vi "3-2 numero di valori casuali generati da RAN - ritardo controllabile da pannello.vi"(4 "stop":bool, 5 "offset":dbl=1.0 format="%.2f", 6 "mult":dbl=100.0 format="%.2f", 7 "ritardo SET":dbl=30.0 format="%.2f") -> (0 "Tempo\ntrascorso":u32, 1 "Ritardo":dbl format="%.2f", 2 "Iterazioni":dbl format="%.2f", 3 "random":dbl format="%.2f")   [LabVIEW 2012]
panel:
  out "random\ngraph":dbl(graph)
  # "Determinare il numero di valori casuali generati da RAN (VI\nche genera un numero compreso tra 1 e 101) \ndall'avvio alla pressione del tasto stop. \n Completare il VI con l'inserzione, nel ciclo di generazione,  di un \nritardo di 30 ms  (controllabile da pannello). Controllare  ciclicamente \n il valore del ritardo generato ed il tempo intercorso tra \n l' avvio del VI e la pressione del tasto Stop."
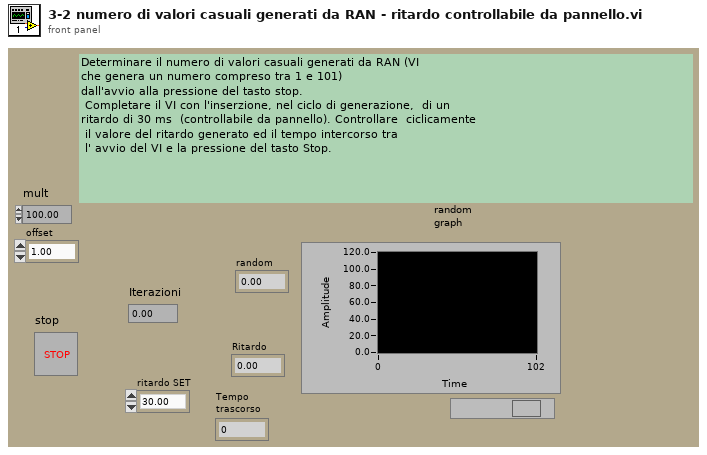
[diagram p1: front panel]
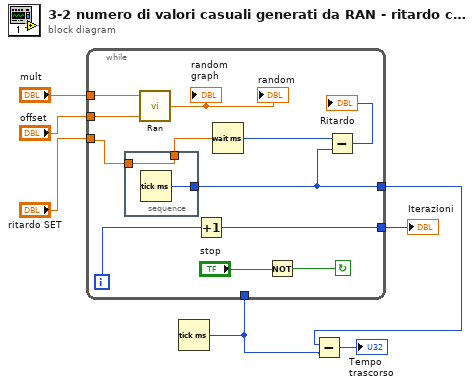
[diagram p0: block diagram]
diagram:
  n1 = Tick Count (ms)() -> (millisecond timer value=w1:u32)
  n2 = while {
    tunnel: [w17] -> w7
    tunnel: "mult" -> [w15]
    tunnel: "offset" -> [w14]
    tunnel: [w10] -> w4
    tunnel: "ritardo SET" -> [w9]
    tunnel: w1 -> [_]
    i -> [w16]
    stop <- w18 continue-if-true
    n3 = stacked-sequence {
      tunnel: [w21] -> w10
      tunnel: w9 -> [w20]
      tunnel: [w20] -> w8
      frame #0 {
        n4 = Tick Count (ms)() -> (millisecond timer value=w21:u32)
      }
    }
    n5 = call "Ran.vi"("offset"=w14, "mul fatt"=w15) -> ("out num"=→"random\ngraph" →"random":dbl)  [unwired: 3 in]
    n6 = Increment(x=w16) -> (x+1=w17:i32)
    n7 = Wait (ms)(milliseconds to wait=w8) -> (millisecond timer value=w12:u32)
    n8 = Not(x="stop") -> (.not. x?=w18:bool)
    n9 = Subtract(x=w12, y=w10) -> (x-y=→"Ritardo":u32)
  }
  "Iterazioni" <- w7
  n10 = Subtract(x=w4, y=w1) -> (x-y=→"Tempo\ntrascorso":u32)
